vi "DcimgToTiff_rach_mod.vi"() -> ()   [LabVIEW 2016]
panel:
  out "Total":i32
  out "Index":i32
  out "Error Out":errorcluster
  out "Total":i32
  out "Index":i32
  in  "DCIMG Path or Folder":path
  # "This is a program to read the images\nwithin a DCIMG file and write them to TIFF files.\nBoth file and folder is OK."
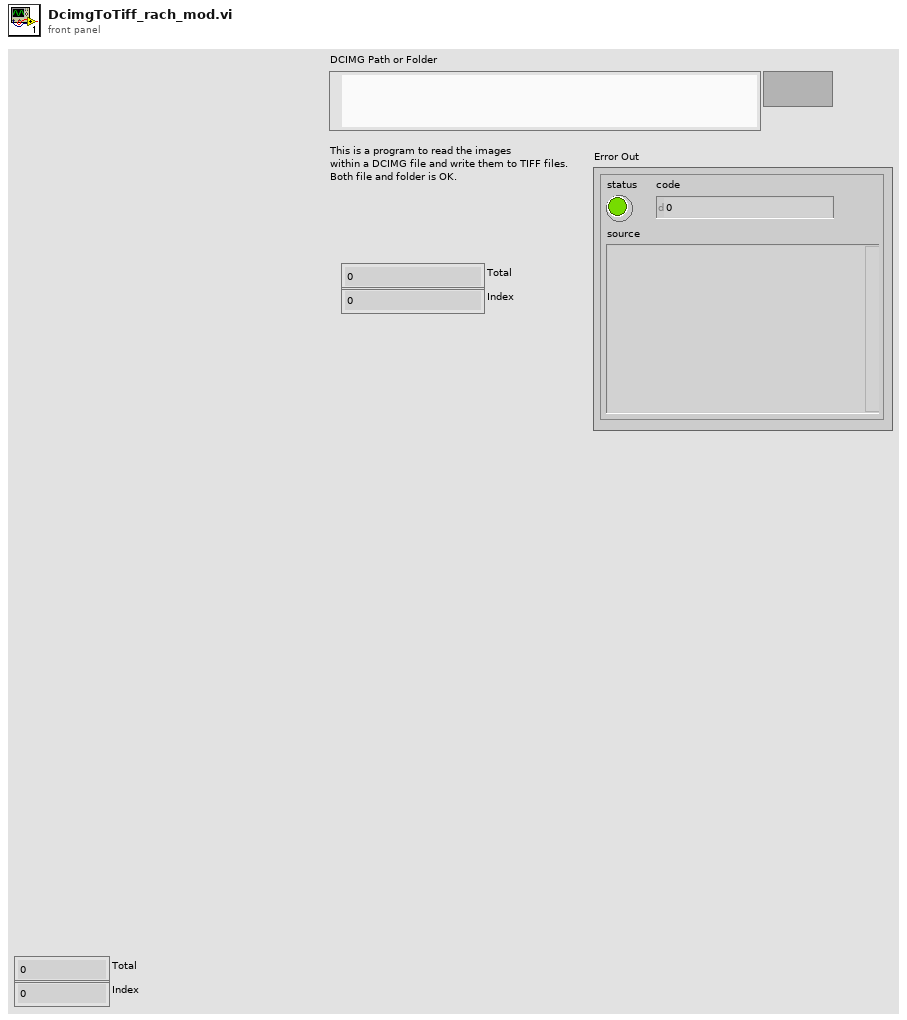
[diagram p1: front panel]
types:
  T1 = typedef "Image Type" = u32
  T2 = typedef "IMAQ Image.ctl" = refnum<image>
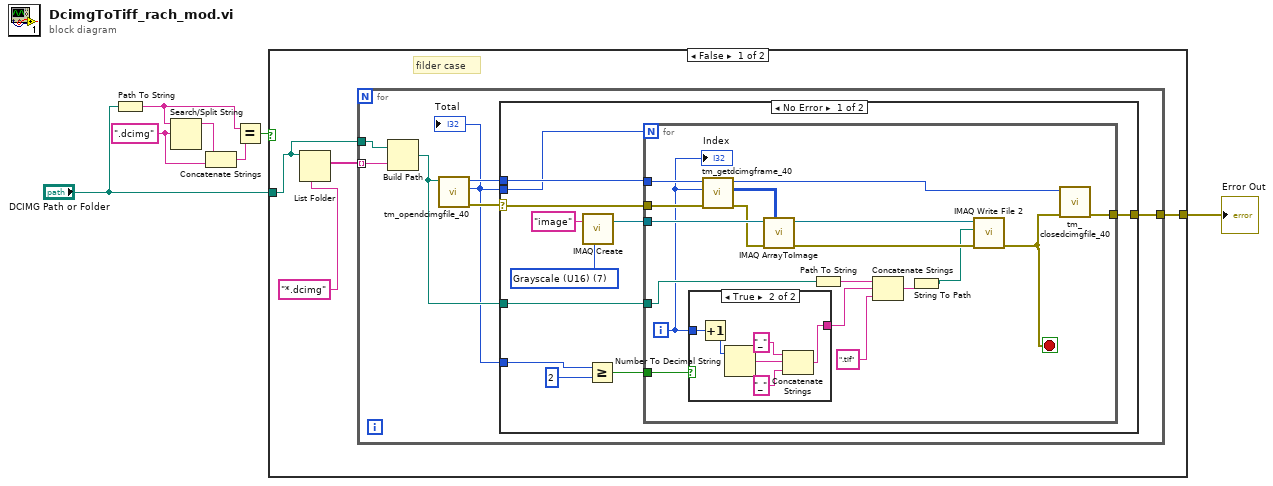
[diagram p0: block diagram]
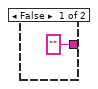
[diagram p2: hidden frame]
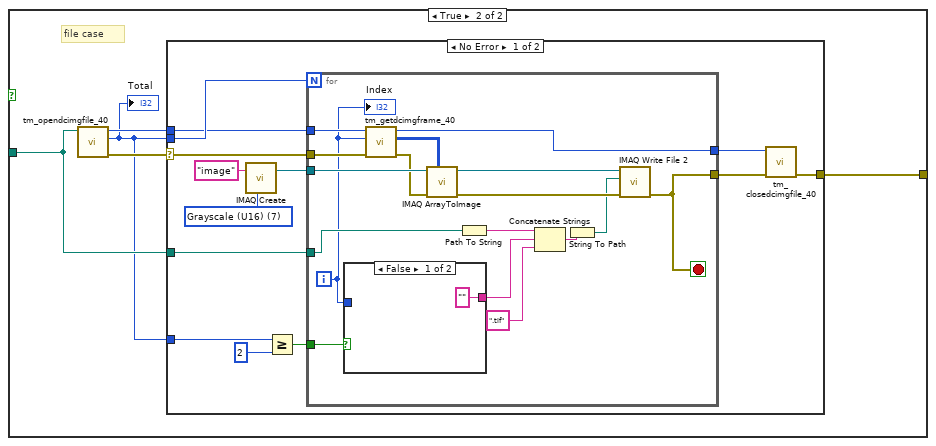
[diagram p4: hidden frame]
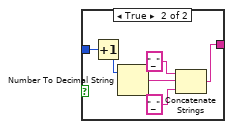
[diagram p5: hidden frame]
diagram:
  w3 = ".dcimg" ("search string/char (-)")
  n1 = Path To String(path="DCIMG Path or Folder") -> (string=w4:string)
  n2 = Search/Split String(string=w4, search string/char (-)=w3) -> (substring before match=w1:string)  [unwired: 1 in, 2 out]
  n3 = Concatenate Strings(w1, w3) -> (w2:string)
  n4 = Equal?(x=w4, y=w2) -> (x = y?=w7:bool)
  n5 = case shown="False" w7 {
    tunnel: "DCIMG Path or Folder" -> [w9 w57]
    tunnel: [w10 w58] -> w5
    frame False {
      # "filder case"
      n6 = List Folder(path=w9, pattern="*.dcimg") -> (filenames=w11:string[])  [unwired: 2 in, 3 out]
      n7 = for {
        tunnel: w11 -> [w17] mode=indexing
        tunnel: [w18] -> w10
        tunnel: w9 -> [w16]
        n8 = Build Path(base path=w16, name or relative path=w17) -> (appended path=w15:path)
        n9 = call <userlib>:"tm_opendcimgfile_40.vi"("Path"=w15) -> ("error out"=w13:errorcluster, "Total Frames"=w12:i32, "File Handle"=w14:u32)  [unwired: 8 in]
        "Total" <- w12
        n10 = case shown="No Error" w13 {
          selector: w13 -> [w21 w55]
          tunnel: [w26 w55] -> w18
          tunnel: w15 -> [w25 _]
          tunnel: w14 -> [w24 _]
          tunnel: w12 -> [w20 _]
          tunnel: w12 -> [w19 _]
          frame No Error {
            w28 = T1 7 items=["Grayscale (U8)", "Grayscale (I16)", "Grayscale (SGL)", "Complex (CSG)", "RGB (U32)", "HSL (U32)", "RGB (U64)", "Grayscale (U16)"] ("Image Type")
            n11 = call "IMAQ Create"("Image Name"="image", "Image Type"=w28) -> ("New Image"=w29:T2)  [unwired: 3 in, 1 out]
            n12 = Greater Or Equal?(x=w19, y=2) -> (x >= y?=w22:bool)
            n13 = for {
              N: w20 -> [_]
              tunnel: w24 -> [w47]
              tunnel: w21 -> [w46]
              tunnel: w29 -> [w45]
              tunnel: w25 -> [w37]
              tunnel: [w34] -> w26
              tunnel: w22 -> [w32]
              i -> [w30]
              stop <- w35 stop-if-true
              n14 = case shown="True" w32 {
                tunnel: ["" w51] -> w31
                tunnel: w30 -> [_ w54]
                frame False {
                }
                frame True {
                  n15 = Increment(x=w54) -> (x+1=w50:i32)
                  n16 = Number To Decimal String(number=w50) -> (decimal integer string=w49:string)  [unwired: 1 in]
                  n17 = Concatenate Strings("_", w49, "_") -> (w51:string)
                }
              }
              n18 = call <userlib>:"tm_getdcimgframe_40.vi"("error in (no error)"=w46, "Frame Index"=w30, "File Handle in"=w47) -> ("error out"=w42:errorcluster, "Data"=w41:u16[][], "File Handle out"=w33:u32)  [unwired: 5 in, 1 out]
              n19 = call "IMAQ ArrayToImage"("Image Pixels (U16)"=w41, "error in (no error)"=w42, "Image"=w45) -> ("error out"=w44:errorcluster, "Image Out"=w43:T2)  [unwired: 7 in]
              n20 = Path To String(path=w37) -> (string=w38:string)
              n21 = Concatenate Strings(w38, w31, ".tif" ("regular expression (\"\")")) -> (w36:string)
              n22 = String To Path(string=w36) -> (path=w39:path)
              n23 = call-poly "IMAQ Write File 2"("error in (no error)"=w44, "File Path"=w39, "Image"=w43) -> ("error out"=w35:errorcluster)  [unwired: 7 in, 1 out]
              n24 = call <userlib>:"tm_closedcimgfile_40.vi"("error in (no error)"=w35, "File Handle"=w33) -> ("error out"=w34:errorcluster)  [unwired: 9 in]
              "Index" <- w30
            }
          }
          frame Error {
          }
        }
      }
    }
    frame True {
      # "file case"
      n25 = call <userlib>:"tm_opendcimgfile_40.vi"("Path"=w57) -> ("error out"=w60:errorcluster, "Total Frames"=w56:i32, "File Handle"=w59:u32)  [unwired: 8 in]
      "Total" <- w56
      n26 = case shown="No Error" w60 {
        selector: w60 -> [w70 w98]
        tunnel: w59 -> [w71 _]
        tunnel: [w73 w98] -> w58
        tunnel: w56 -> [w72 _]
        tunnel: w57 -> [w64 _]
        tunnel: w56 -> [w61 _]
        frame No Error {
          w68 = T1 7 items=["Grayscale (U8)", "Grayscale (I16)", "Grayscale (SGL)", "Complex (CSG)", "RGB (U32)", "HSL (U32)", "RGB (U64)", "Grayscale (U16)"] ("Image Type")
          n27 = call "IMAQ Create"("Image Name"="image", "Image Type"=w68) -> ("New Image"=w67:T2)  [unwired: 3 in, 1 out]
          n28 = Greater Or Equal?(x=w61, y=2) -> (x >= y?=w63:bool)
          n29 = for {
            N: w72 -> [_]
            tunnel: w71 -> [w90]
            tunnel: w70 -> [w89]
            tunnel: w67 -> [w88]
            tunnel: [w82] -> w65
            tunnel: [w84] -> w66
            tunnel: w64 -> [w79]
            tunnel: w63 -> [w74]
            i -> [w75]
            stop <- w82 stop-if-true
            n30 = case shown="False" w74 {
              tunnel: ["" w94] -> w76
              tunnel: w75 -> [_ w97]
              frame False {
              }
              frame True {
                n31 = Increment(x=w97) -> (x+1=w93:i32)
                n32 = Number To Decimal String(number=w93) -> (decimal integer string=w92:string)  [unwired: 1 in]
                n33 = Concatenate Strings("_", w92, "_") -> (w94:string)
              }
            }
            n34 = call <userlib>:"tm_getdcimgframe_40.vi"("error in (no error)"=w89, "Frame Index"=w75, "File Handle in"=w90) -> ("error out"=w85:errorcluster, "Data"=w83:u16[][], "File Handle out"=w84:u32)  [unwired: 5 in, 1 out]
            n35 = call "IMAQ ArrayToImage"("Image Pixels (U16)"=w83, "error in (no error)"=w85, "Image"=w88) -> ("error out"=w87:errorcluster, "Image Out"=w86:T2)  [unwired: 7 in]
            n36 = Path To String(path=w79) -> (string=w80:string)
            n37 = Concatenate Strings(w80, w76, ".tif" ("regular expression (\"\")")) -> (w78:string)
            n38 = String To Path(string=w78) -> (path=w77:path)
            n39 = call-poly "IMAQ Write File 2"("error in (no error)"=w87, "File Path"=w77, "Image"=w86) -> ("error out"=w82:errorcluster)  [unwired: 7 in, 1 out]
            "Index" <- w75
          }
          n40 = call <userlib>:"tm_closedcimgfile_40.vi"("error in (no error)"=w65, "File Handle"=w66) -> ("error out"=w73:errorcluster)  [unwired: 9 in]
        }
        frame Error {
        }
      }
    }
  }
  "Error Out" <- w5
